vi "Explode String.vi"(7 "Delimiter (Comma)":string=",", 11 "Delimited String":string) -> (3 "String Array":string[](array[string]))   [LabVIEW 2020, in "Better Search.lvlib"]
uses:
  Better Search.lvlib
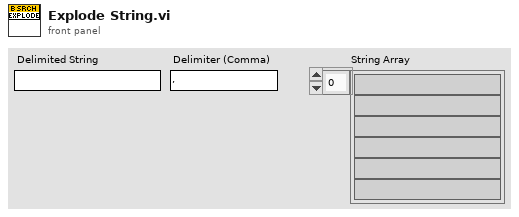
[diagram p1: front panel]
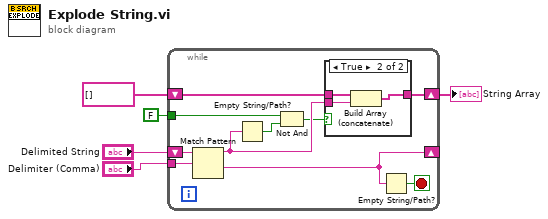
[diagram p0: block diagram]
diagram:
  n1 = while {
    tunnel: "Delimiter (Comma)" -> [w14]
    shift-right: [w11] -> _
    shift-left: "Delimited String" -> [w15]
    shift-right: [w12] -> w2
    shift-left: string[] [] -> [w10]
    tunnel: FALSE ("Remove Empty? (F)") -> [w7]
    stop <- w13 stop-if-true
    n2 = Match Pattern(string=w15, regular expression=w14) -> (before substring=w9:string, after substring=w11:string)  [unwired: 1 in, 2 out]
    n3 = Empty String/Path?(string/path=w9) -> (empty?=w8:bool)
    n4 = Not And(1:w8, 2:w7) -> (0:w6:bool)
    n5 = case shown="True" w6 {
      tunnel: [w16 w19] -> w12
      tunnel: w10 -> [w16 w18]
      tunnel: w9 -> [_ w17]
      frame False {
      }
      frame True {
        n6 = Build Array (concatenate)(w18, w17) -> (w19:string[])
      }
    }
    n7 = Empty String/Path?(string/path=w11) -> (empty?=w13:bool)
  }
  "String Array" <- w2
